vi "LVClass_WavefrontCorrectorSet Get Parameter Real Default Value.vi"(0 "WavefrontCorrectorSet in":refnum<class "WavefrontCorrectorSet.lvclass">, 5 "parameter_name":string, 11 "error in (no error)":errorcluster) -> (4 "WavefrontCorrectorSet out":refnum<class "WavefrontCorrectorSet.lvclass">, 6 "defaultValue":dbl, 15 "error out":errorcluster)   [LabVIEW 2020, in "WavefrontCorrectorSet.lvclass"]
doc: "WavefrontCorrector parameter default value getter for parameter of type float.\n\n--------------------------------------------------------------------------------\n\n<B>wavefrontcorrector_setIn </B> : WavefrontCorrectorSet object.\n<B>wavefrontcorrector_setOut </B> : WavefrontCorrectorSet object.\n<B>parameter_name </B> : Parameter name.\n<B>default_value </B> : Parameter default value.\n<B>ErrorIn </B> : Error\n<B>ErrorOut </B> : Error\n\n--------------------------------------------------------------------------------"
uses:
  WavefrontCorrectorSet.lvclass
  WavefrontCorrectorSet.lvclass/WavefrontCorrectorSet.ctl
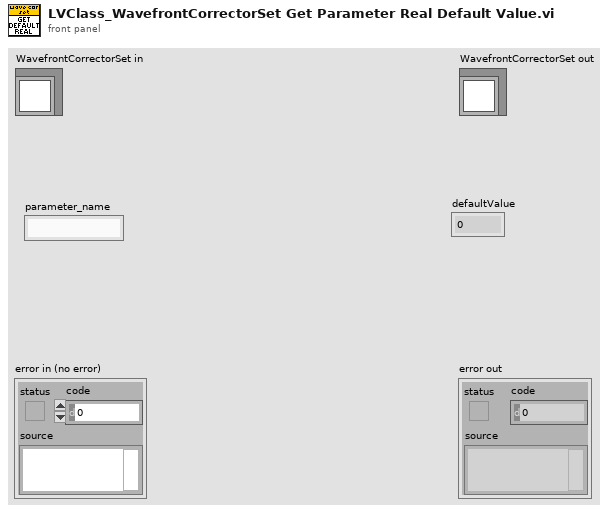
[diagram p1: front panel]
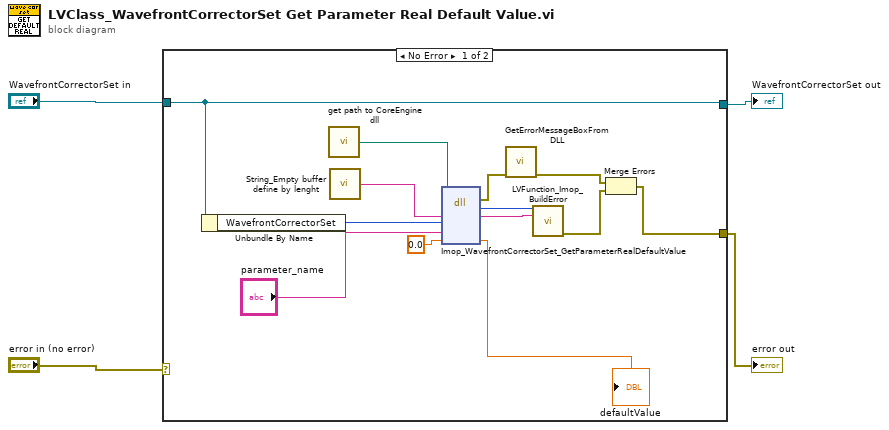
[diagram p0: block diagram]
diagram:
  n1 = case shown="No Error" "error in (no error)" {
    selector: "error in (no error)" -> [_ w18]
    tunnel: "WavefrontCorrectorSet in" -> [w9 w19]
    tunnel: [w9 w19] -> w1
    tunnel: [w6 w18] -> w2
    frame No Error {
      n2 = Unbundle By Name(w9) -> ("WavefrontCorrectorSet"=w8:i32)
      n3 = call "get path to CoreEngine dll.vi"() -> ("path to c_interface_vc100.dll"=w12:path)  [unwired: 12 in, 3 out]
      n4 = call "String_Empty buffer define by lenght.vi"() -> ("Empty buffer"=w15:string)  [unwired: 1 in]
      n5 = dll-call lib="D:/soft/HASO_v3/C_interface/Sources/Build/vc100/Release/c_interface_vc100.dll" fn="Imop_WavefrontCorrectorSet_GetParameterRealDefaultValue"(path in=w12, "message"=w15, "objet"=w8, "parameter_name"="parameter_name", "defaultValue"=0.0 ("min")) -> (error out=w11:errorcluster, "return type"=w17:i32, "message"=w16:string, "defaultValue"=→"defaultValue":dbl)  [unwired: 4 in, 1 out]
      n6 = call "GetErrorMessageBoxFromDLL.vi"("error IN"=w11) -> ("error OUT"=w5:errorcluster)  [unwired: 10 in]
      n7 = call "LVFunction_Imop_BuildError.vi"("code"=w17, "String to Prepend to source (\"\")"=w16) -> ("error out"=w7:errorcluster)  [unwired: 13 in]
      n8 = Merge Errors(w5, w7) -> (w6:errorcluster)
    }
    frame Error {
    }
  }
  "error out" <- w2
  "WavefrontCorrectorSet out" <- w1
